vi "Belkin Polar to Complex.vi"() -> ()   [LabVIEW 2015]
uses:
  Controls/FPGA Scanner State.ctl
  <vilib>/Platform/TimedLoop/XDataNode/timing_clust.ctl
  <vilib>/Platform/TimedLoop/XDataNode/nitl_modes.ctl
  <vilib>/Platform/TimedLoop/XDataNode/wakeup.ctl
  <vilib>/rvi/FXPMathLib/FxpPolarToRect/subVIs/nifxpmath_PolarToRect_SimConfig.ctl
  <vilib>/rvi/Emulation/niFpgaGetClockAttributes.vi
  <vilib>/rvi/Emulation/niFpgaSctlEmulationGetInTimedLoop.vi
  <vilib>/rvi/Emulation/niFpgaEmulationReportErrorSimple.vi
  <vilib>/rvi/Emulation/niFpgaProcessEmulError.vi
  <vilib>/rvi/eio/common/nirviEmuTemplateMethod_errors.vi
  <vilib>/rvi/Emulation/niFpgaCriticalErrorInLSC.vi
  <vilib>/rvi/FXPMathLib/FxpPolarToRect/simVIs/DllFxpPolarToRectTemp_sub.vi
  <vilib>/eio/EIONode/EIONode.xnode
  <vilib>/Platform/TimedLoop/XDataNode/XDataNode.xnode
  <vilib>/rvi/FXPMathLib/FxpPolarToRect/XNode/nifxpmath_PolarToRect.xnode
  <vilib>/rvi/FXPMathLib/FxpMul/XNode/nifxpmath_Multiplier.xnode
  <vilib>/rvi/FXPMathLib/FxpAdd/XNode/nifxpmath_Add.xnode
  <vilib>/Platform/TimedLoop/XDataNode/XDNodeRunTimeDep.lvlib
  <vilib>/rvi/FXPMathLib/sim/FxpSim.dll
panel:
  in  "EngleDelta":fxp<+/-,16,1>
  in  "EndEngle":fxp<+/-,16,1>
  in  "StartAngle":fxp<+,16,1>
  in  "ScanOnce":bool
  in  "ScanContinues":bool
  in  "ManLaser":bool
  out "LaserEn":bool
  out "ScanState":T1
  in  "ManAngle":fxp<+,16,1>
  in  "Decimator":u16
  out "Yscan":fxp<+/-,35,5>
  out "Xscan":fxp<+/-,35,5>
  in  "Ypos":fxp<+/-,16,1>
  in  "Xpos":fxp<+/-,16,1>
  in  "Yofset":fxp<+/-,16,1>
  in  "Xofset":fxp<+/-,16,1>
  in  "Ygain":fxp<+/-,16,1>=0.999969482421875
  in  "Xgain":fxp<+/-,16,1>=0.999969482421875
  out "Yout":fxp<+/-,17,2>
  out "Xout":fxp<+/-,17,2>
  in  "PupilRadius":fxp<+,15,0>
  in  "ScanAngle":fxp<+,16,1>
  # "Calibration"
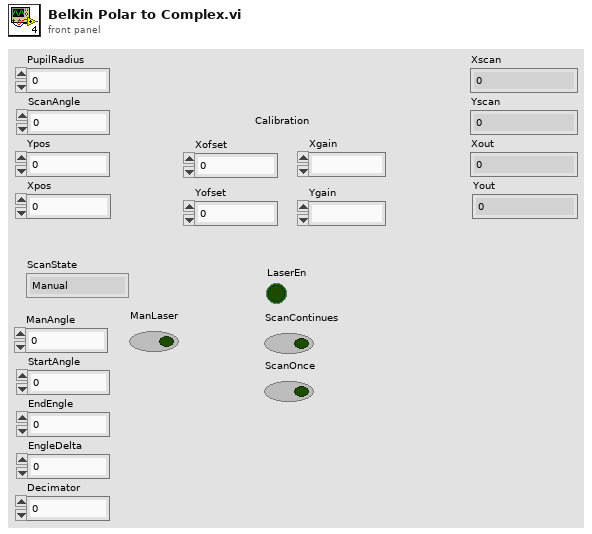
[diagram p1: front panel]
types:
  T1 = typedef "FPGA Scanner State.ctl" = enum16{"Manual", "GOTO Start", "GOTO next", "Laser OFF"}
  T2 = typedef "XDNodeRunTimeDep.lvlib/timing_clust.ctl" = cluster{"Expected End [f-1]":u64, "Actual End [f-1]":u64, "Finished Late? [f-1]":bool, "Expected End [i-1]":u64, "Actual End [i-1]":u64, "Finished Late? [i-1]":bool, "Expected Start [i]":u64, "Actual Start [i]":u64, "Expected Start [f]":u64, "Actual Start [f]":u64, "Source Name":string, "Structure Name":string, "Period":i64, "Deadline":i64, "Offset":i64, "Start":i64, "Priority":i32, "Timeout":i32, "Mode":T3, "Wakeup Reason":T4, "Error":errorcluster, "Source Type":string, "Secondary Source Type":string, "Global End Time":u64, "Global Start Time":u64, "Frame Duration":u64, "Iteration Duration":u64, "Assigned CPU":i32, "I/O Scan Engine Mode":u32}
  T3 = typedef "XDNodeRunTimeDep.lvlib/nitl_modes.ctl" = enum32{"No Change", "Process missed periods, maintain original phase", "Discard missed periods, maintain original phase", "Process missed periods, ignore original phase", "Discard missed periods, ignore original phase"}
  T4 = typedef "XDNodeRunTimeDep.lvlib/wakeup.ctl" = enum32{"Normal", "Aborted", "Asynchronous wakeup", "Timing source error", "Timed loop error", "Timeout"}
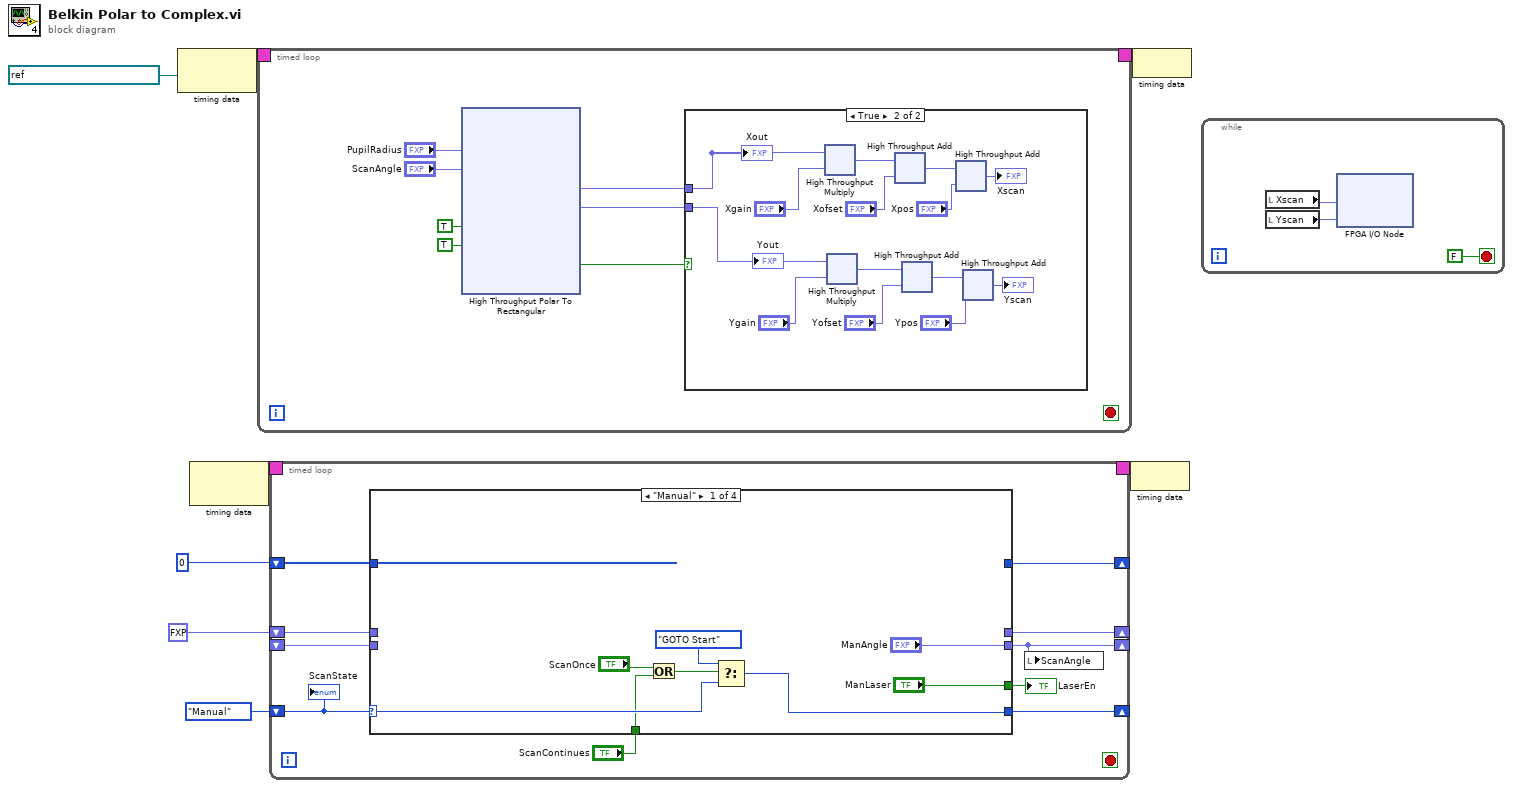
[diagram p0: block diagram]
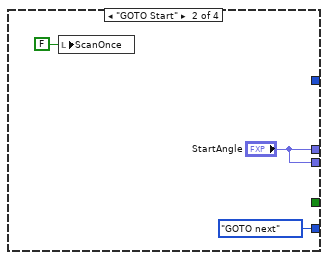
[diagram p2: hidden frame]
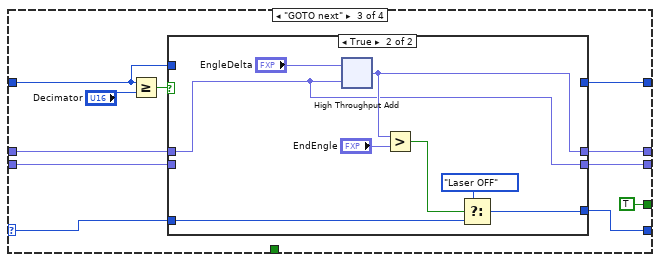
[diagram p3: hidden frame]
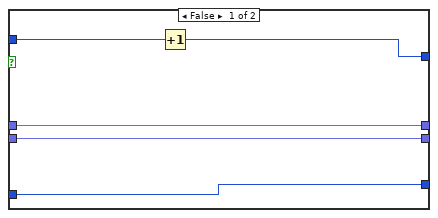
[diagram p4: hidden frame]
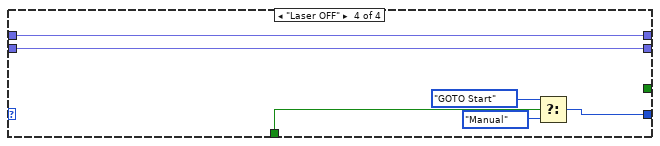
[diagram p5: hidden frame]
diagram:
  n1 = node-c288(refnum<k21> "40 MHz Onboard Clock" ("Source Name")) -> (w8:T2)
  n2 = node-c288() -> (w5:T2)  [unwired: 1 in]
  n3 = timed-loop {
    timing: w8 -> [_]
    timing-out: [_] -> w7
    stop <- _ stop-if-true
    n4 = xnode "High Throughput Polar To Rectangular"("magnitude"="PupilRadius", "phase (pi)"="ScanAngle", "input valid"=TRUE, "ready for output (T)"=TRUE) -> ("x"=w13:fxp<+/-,17,2>, "y"=w12:fxp<+/-,17,2>, "output valid"=w9:bool)  [unwired: 1 out]
    n5 = case shown="True" w9 {
      tunnel: w13 -> [_ w29]
      tunnel: w12 -> [_ w28]
      frame False {
      }
      frame True {
        n6 = xnode ("High Throughput Multiply")("x"=w29, "y"="Xgain") -> ("x*y"=w25:fxp<+/-,33,3>)
        n7 = xnode ("High Throughput Multiply")("x"=w28, "y"="Ygain") -> ("x*y"=w24:fxp<+/-,33,3>)
        n8 = xnode ("High Throughput Add")("x"=w25, "y"="Xofset") -> ("x+y"=w21:fxp<+/-,34,4>)
        n9 = xnode ("High Throughput Add")("x"=w24, "y"="Yofset") -> ("x+y"=w19:fxp<+/-,34,4>)
        n10 = xnode ("High Throughput Add")("x"=w21, "y"="Xpos") -> ("x+y"=→"Xscan":fxp<+/-,35,5>)
        n11 = xnode ("High Throughput Add")("x"=w19, "y"="Ypos") -> ("x+y"=→"Yscan":fxp<+/-,35,5>)
        "Xout" <- w29
        "Yout" <- w28
      }
    }
  }
  n12 = timed-loop {
    timing: w5 -> [_]
    timing-out: [_] -> w4
    shift-right: [w78] -> _
    shift-left: u16 0 -> [w79]
    shift-right: [w75] -> _
    shift-left: FPGA_Scanner_State."Manual" -> [w77]
    shift-right: [w74] -> _
    shift-left: fxp<+,16,1> 0.0 ("x+y") -> [w73]
    shift-right: [w71] -> _
    shift-left: _ -> [w72]
    stop <- _ stop-if-true
    n13 = case shown="\"Manual\"" w77 {
      selector: w77 -> [w83 _ w95 _]
      tunnel: w79 -> [_ _ w100 _]
      tunnel: [_ _ w99 _] -> w78
      tunnel: ["ManLaser" _ TRUE ("ManLaser") _] -> w76
      tunnel: [w82 FPGA_Scanner_State."GOTO next" w94 w115] -> w75
      tunnel: [_ "StartAngle" w96 w119] -> w74
      tunnel: w73 -> [_ _ w97 w119]
      tunnel: ["ManAngle" "StartAngle" w92 w120] -> w71
      tunnel: w72 -> [_ _ w91 w120]
      tunnel: "ScanContinues" -> [w80 _ _ w118]
      frame "Manual" {
        n14 = Or(x="ScanOnce", y=w80) -> (x .or. y?=w85:bool)
        n15 = Select(t=FPGA_Scanner_State."GOTO Start", s=w85, f=w83) -> (s? t:f=w82:T1)
      }
      frame "GOTO Start" {
        n16 = local write "ScanOnce"(FALSE ("ScanOnce")) -> ()
      }
      frame "GOTO next" {
        n17 = Greater Or Equal?(x=w100, y="Decimator") -> (x >= y?=w101:bool)
        n18 = case shown="True" w101 {
          tunnel: w100 -> [w106 _]
          tunnel: [w104 _] -> w99
          tunnel: w97 -> [w105 w107]
          tunnel: [w105 w113] -> w96
          tunnel: w95 -> [w102 w110]
          tunnel: [w102 w108] -> w94
          tunnel: [w103 w107] -> w92
          tunnel: w91 -> [w103 _]
          frame False {
            n19 = Increment(x=w106) -> (x+1=w104:u16)
          }
          frame True {
            n20 = xnode ("High Throughput Add")("x"="EngleDelta", "y"=w107) -> ("x+y"=w113:fxp<+,16,1>)
            n21 = Greater?(x=w113, y="EndEngle") -> (0:w111:bool)
            n22 = Select(t=FPGA_Scanner_State."Laser OFF", s=w111, f=w110) -> (s? t:f=w108:T1)
          }
        }
      }
      frame "Laser OFF" {
        n23 = Select(t=FPGA_Scanner_State."GOTO Start", s=w118, f=FPGA_Scanner_State."Manual") -> (s? t:f=w115:T1)
      }
    }
    "LaserEn" <- w76
    n24 = local write "ScanAngle"(w71) -> ()
    "ScanState" <- w77
  }
  n25 = node-c288(w4) -> ()
  n26 = node-c288(w7) -> ()
  n27 = while {
    stop <- FALSE stop-if-true
    n28 = local read "Xscan"() -> (w124:fxp<+/-,35,5>)
    n29 = local read "Yscan"() -> (w123:fxp<+/-,35,5>)
    n30 = xnode "FPGA I/O Node"("ScanX"=w124, "ScanY"=w123) -> ()  [unwired: 2 in, 2 out]
  }
